vi "Simulador Circuito RLC.vi"() -> ()   [LabVIEW 2020]
uses:
  <vilib>/measure/NI_MABase.lvlib
panel:
  in  "Duty Cicle":dbl
  in  "Informação da amostragem":T1={"Taxa de amostragem"=1000.0, "N° de amostras"=10000.0} {"N° de amostras" format="%#.6g"; "Taxa de amostragem" format="%#.6g"}
  in  "C":dbl
  in  "L":dbl
  in  "R":dbl
  in  "Gerar ondas\nde saída":bool
  in  "Gerar onda \nde Entrada":bool
  in  "Tipo de Onda":u16(ring) items=["Onda qualquer", "Senoidal", "Quadrada", ""]
  out "Corrente":dbl(graph)
  out "Tensão no capacitor":dbl(graph)
  out "Onda de Entrada":waveform(dbl)(graph)
  in  "Amplitude":dbl
  in  "Frequência":dbl
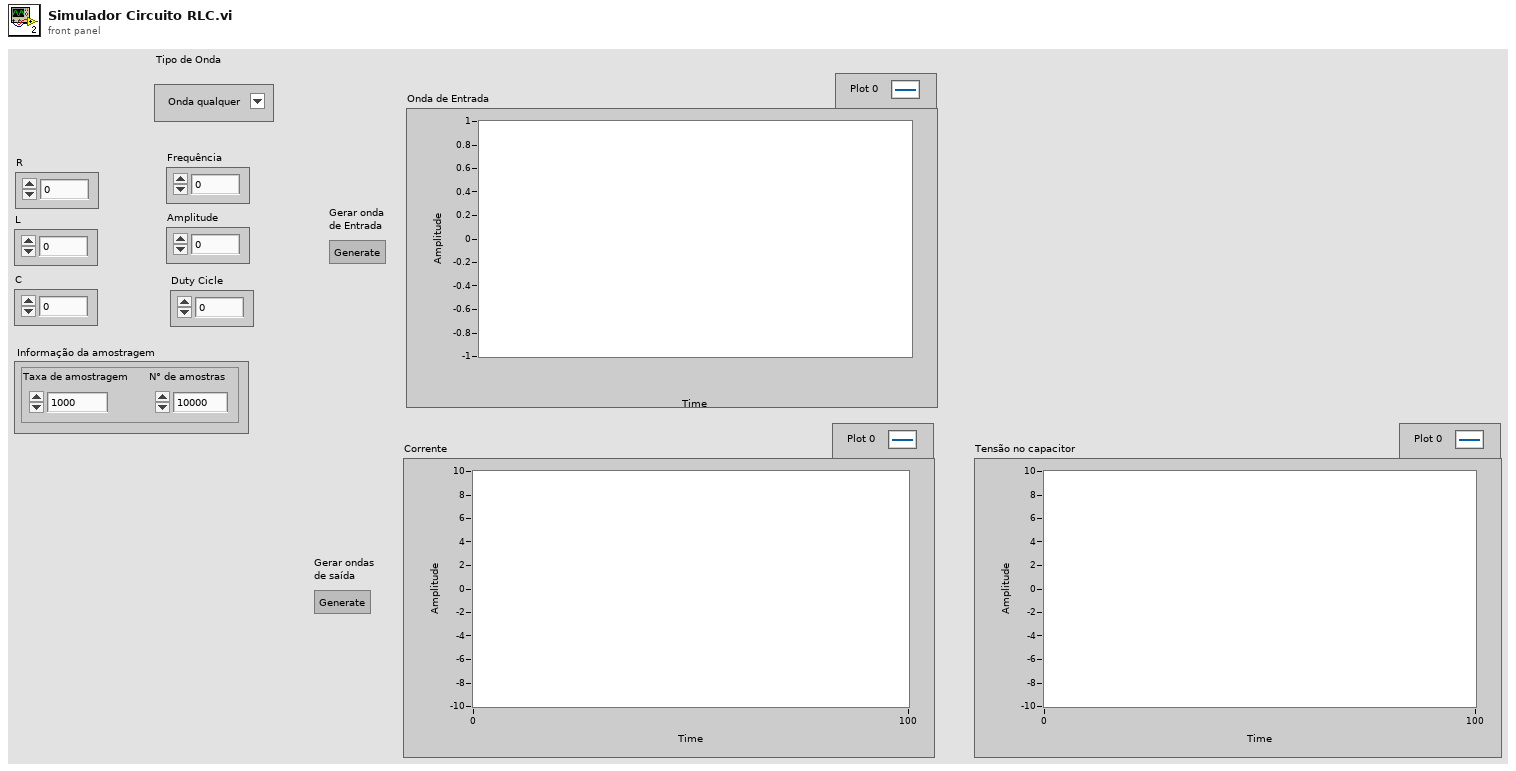
[diagram p1: front panel]
types:
  T1 = cluster{"Taxa de amostragem":dbl, "N° de amostras":dbl}
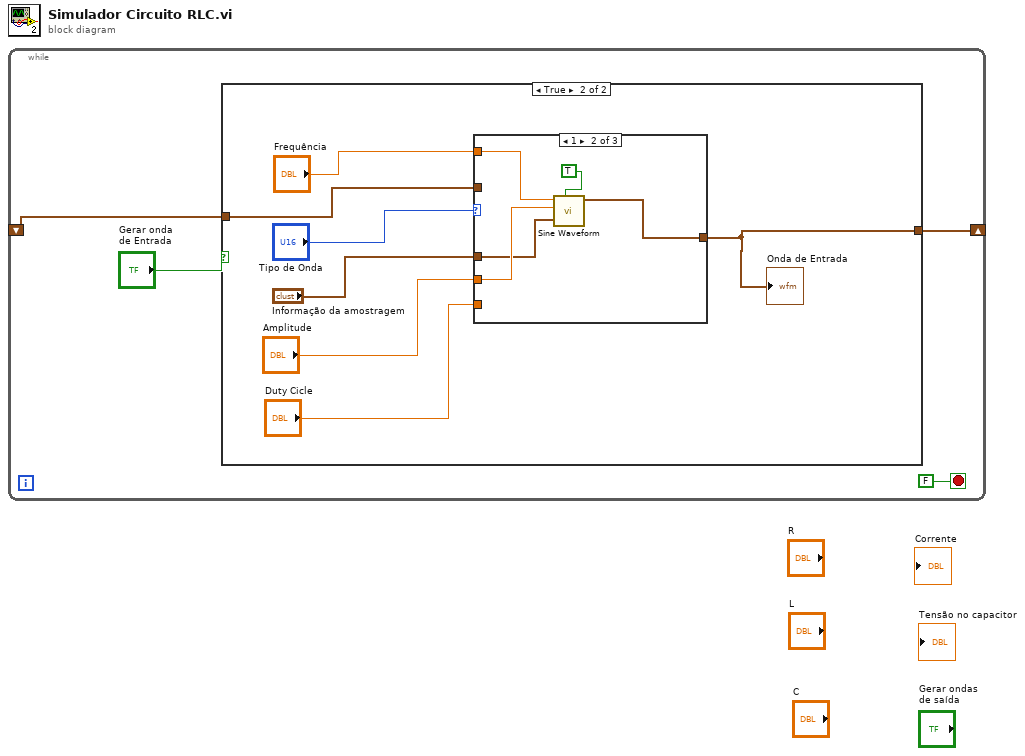
[diagram p0: block diagram]
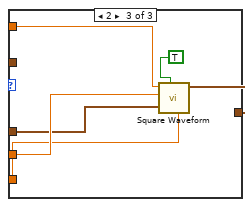
[diagram p4: hidden frame]
diagram:
  n1 = while {
    shift-right: [w2] -> _
    shift-left: _ -> [w3]
    stop <- FALSE stop-if-true
    n2 = case shown="True" "Gerar onda \nde Entrada" {
      tunnel: w3 -> [w5 w10]
      tunnel: [w5 w9] -> w2
      frame False {
      }
      frame True {
        n3 = case shown="1" "Tipo de Onda" {
          tunnel: "Amplitude" -> [_ w17 w23]
          tunnel: "Frequência" -> [_ w18 w24]
          tunnel: w10 -> [w13 _ _]
          tunnel: "Informação da amostragem" -> [_ w16 w22]
          tunnel: [w13 w15 w20] -> w9
          tunnel: "Duty Cicle" -> [_ _ w21]
          frame Default {
          }
          frame 1 {
            n4 = call <vilib>:"Sine Waveform.vi"("sampling info"=w16, "reset signal"=TRUE, "amplitude"=w17, "frequency"=w18) -> ("signal out"=w15:waveform(dbl))  [unwired: 6 in, 1 out]
          }
          frame 2 {
            n5 = call <vilib>:"Square Waveform.vi"("duty cycle (%)"=w21, "sampling info"=w22, "reset signal"=TRUE, "amplitude"=w23, "frequency"=w24) -> ("signal out"=w20:waveform(dbl))  [unwired: 5 in, 1 out]
          }
        }
        "Onda de Entrada" <- w9
      }
    }
  }
